vi "message handler main.vi"(11 "messageHandler":T2 {"params"."controlChannels"."ballControl" items=["Module6/output0", "Module6/output1", "Module6/output2", "Module6/output3", "Not-Used"]; "params"."controlChannels"."butterflyControl" items=["Module6/output0", "Module6/output1", "Module6/output2", "Module6/output3", "Not-Used"]; "params"."controlChannels"."speedControl" items=["Module6/output0", "Module6/output1", "Module6/output2", "Module6/output3", "Not-Used"]}) -> ()   [LabVIEW 2018]
uses:
  supporting VIs/polymorphic VIs/enqueue for data stream.vi
  supporting VIs/polymorphic VIs/enqueue for comms.vi
  supporting VIs/polymorphic VIs/enqueue for user interface.vi
  RT/Type Defs/RT Status.ctl
  supporting VIs/polymorphic VIs/enqueue for custom.vi
  supporting VIs/polymorphic VIs/release message handler queue.vi
  supporting VIs/polymorphic VIs/enqueue for message handler.vi
  supporting VIs/polymorphic VIs/de-queue for message handler.vi
  supporting VIs/polymorphic VIs/enqueue for data processor.vi
  comms loop/delayedMessages/delayedMessageHandler.vi
  customVI/liveData/state.ctl
  type defs/message handler data.ctl
panel:
  out "RT status":T1
  out "commands":string[](array[string])
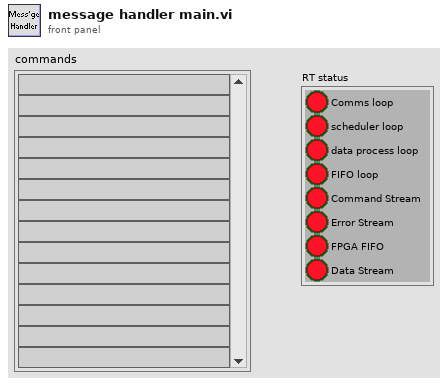
[diagram p1: front panel]
types:
  T1 = typedef "RT Status.ctl" = cluster{"Comms loop":bool, "scheduler loop":bool, "data process loop":bool, "FIFO loop":bool, "Command Stream":bool, "Error Stream":bool, "FPGA FIFO":bool, "Data Stream":bool}
  T2 = typedef "message handler data.ctl" = cluster{"params":cluster{"configFileID":u32, "configFilePath":path, "channelConfigFilePath":path, "incidentLogfile":path, "controlChannels":cluster{"ballControl":u16, "butterflyControl":u16, "speedControl":u16}, "pulsatorVIPath":path, "customVIPath":path, "HowdenAir":cluster{"vent Howden":bool, "Howden%":dbl}}, "vars":cluster{"commsStatus":bool[], "controlIndex":cluster{"ballControl":u16, "butterflyControl":u16, "speedControl":u16}, "customVIRef":refnum<vi>, "Interlocks":cluster{"gearboxOil":bool, "bearingOil":bool, "gearboxAir":bool}, "motorRunning":bool, "liveDataQ":refnum<queue>[]}}
  T3 = typedef "Queues.ctl" = cluster{"messageHandler":refnum<queue>, "comms":refnum<queue>, "dataStream":refnum<queue>, "dataProcessor":refnum<queue>, "fileIO":refnum<queue>, "userInterface":refnum<queue>, "errors":refnum<queue>, "customCompressor":refnum<queue>}
  T4 = cluster{"gearboxOil":bool, "bearingOil":bool, "gearboxAir":bool}
  T5 = typedef "state.ctl" = enum16{"readData", "init", "channel", "mode", "quit"}
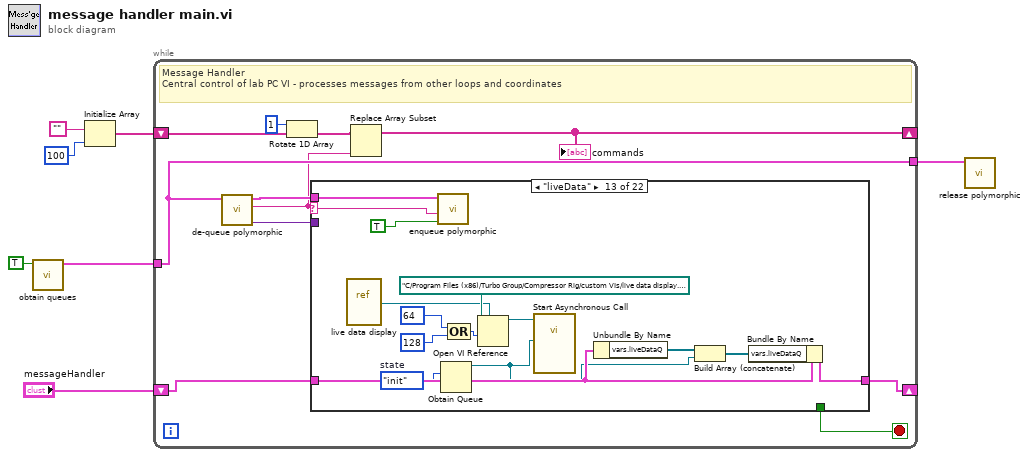
[diagram p0: block diagram]
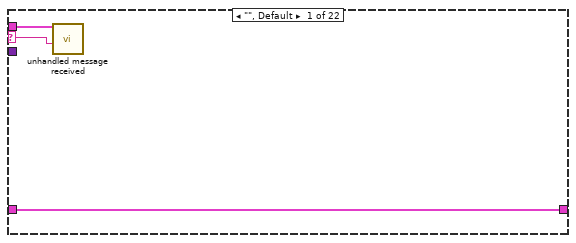
[diagram p2: hidden frame]
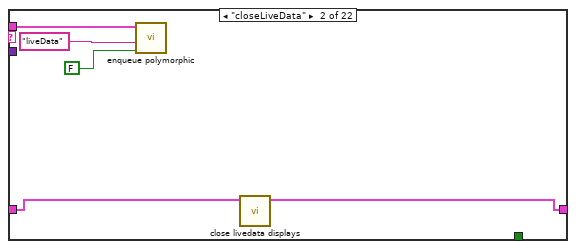
[diagram p3: hidden frame]
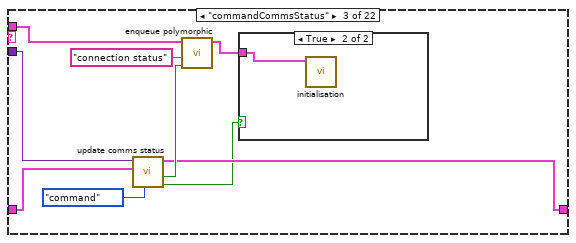
[diagram p4: hidden frame]
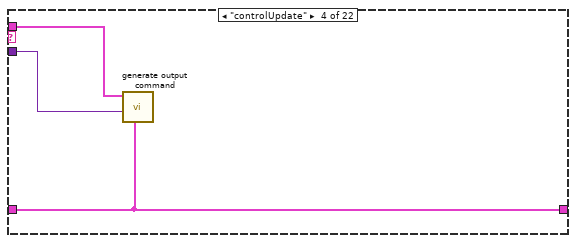
[diagram p6: hidden frame]
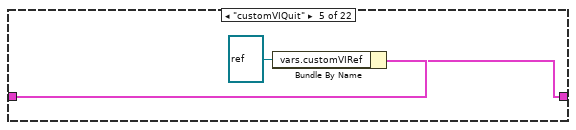
[diagram p7: hidden frame]
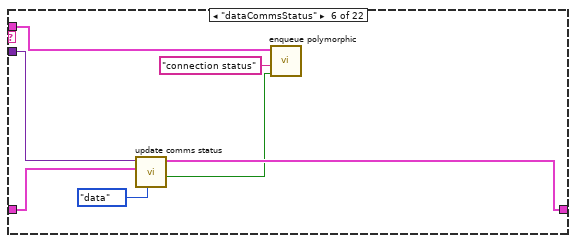
[diagram p8: hidden frame]
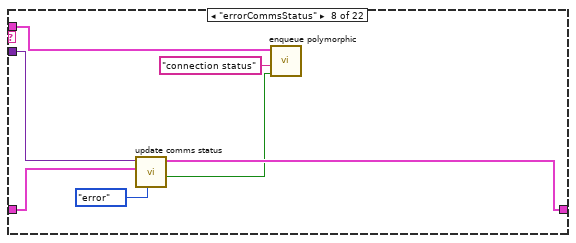
[diagram p10: hidden frame]
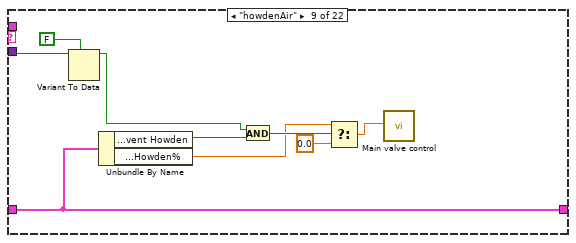
[diagram p11: hidden frame]
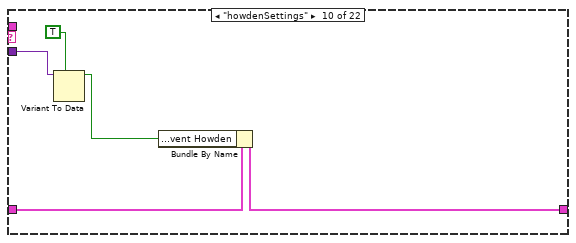
[diagram p12: hidden frame]
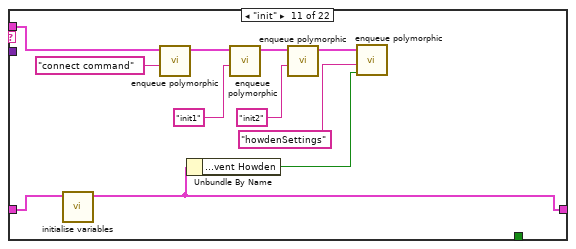
[diagram p13: hidden frame]
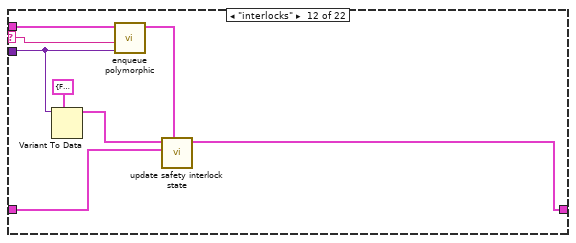
[diagram p14: hidden frame]
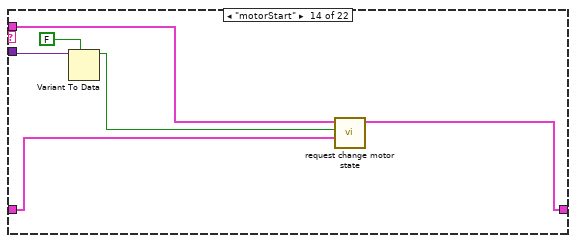
[diagram p15: hidden frame]
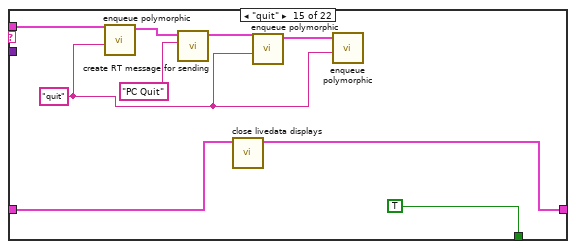
[diagram p16: hidden frame]
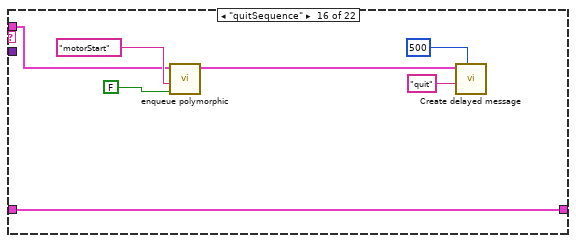
[diagram p17: hidden frame]
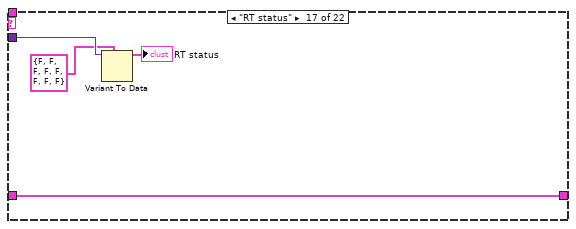
[diagram p18: hidden frame]
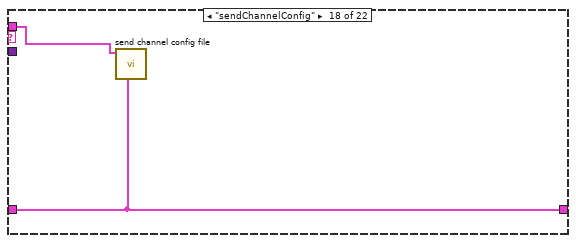
[diagram p19: hidden frame]
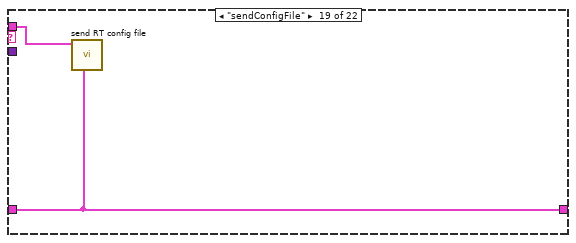
[diagram p20: hidden frame]
diagram:
  n1 = call "obtain queues.vi"("initialise? (F)"=TRUE) -> ("queues"=w7:T3)  [unwired: 10 in]
  n2 = Initialize Array("", 100 ("dimension size")) -> (w3:string[])
  n3 = while {
    tunnel: w7 -> [w15]
    tunnel: [w15] -> w6
    shift-right: [w14] -> _
    shift-left: "messageHandler" -> [w13]
    shift-right: [w9] -> _
    shift-left: w3 -> [w12]
    stop <- w17 stop-if-true
    # "Message Handler\nCentral control of lab PC VI - processes messages from other loops and coordinates"
    n4 = call-poly "de-queue polymorphic.vi"("Queues"=w15) -> ("data"=w18:variant, "message"=w8:string, "Queues out"=w16:T3)  [unwired: 8 in]
    n5 = Rotate 1D Array(1:w12, 2:1 ("n")) -> (0:w10:string[])
    n6 = case shown="\"liveData\"" w8 {
      selector: w8 -> [w19 _ _ _ _ _ _ _ _ _ _ w88 w100 _ _ _ _ _ _ _ _ _]
      tunnel: w18 -> [_ _ w34 w38 _ w47 _ w55 w66 w69 _ w86 _ w111 _ _ w131 _ _ _ w141 _]
      tunnel: [_ _ _ _ _ _ _ _ _ _ _ _ _ _ TRUE _ _ _ _ _ _ _] -> w17
      tunnel: w16 -> [w20 w26 w32 w39 _ w45 _ w53 _ _ w80 w89 w101 w109 w114 w125 _ w133 w135 w138 w140 _]
      tunnel: [w21 w24 w28 w37 w41 w48 w50 w56 w64 w70 w73 w87 w98 w107 w112 w124 w128 w132 w134 w136 w139 w142] -> w14
      tunnel: w13 -> [w21 w25 w35 w37 w42 w49 w50 w57 w64 w71 w82 w90 w99 w108 w113 w124 w128 w132 w134 w137 w139 w142]
      frame "", Default {
        n7 = call "unhandled message received.vi"("unhandledMessage"=w19, "queues"=w20) -> ()  [unwired: 10 in]
      }
      frame "closeLiveData" {
        n8 = call-poly "enqueue polymorphic.vi"("data"=FALSE, "message"="liveData", "Queues"=w26) -> ()  [unwired: 8 in, 1 out]
        n9 = call "close livedata displays.vi"("messageHandler in"=w25) -> ("messageHandler out"=w24:T2)  [unwired: 10 in]
      }
      frame "commandCommsStatus" {
        n10 = call "update comms status.vi"("comms"=enum16{"command", "error", "data"}."command", "messageHandler in"=w35, "data"=w34) -> ("this comms"=w27:bool, "connection status"=w30:bool, "messageHandler out"=w28:T2)  [unwired: 6 in]
        n11 = call-poly "enqueue polymorphic.vi"("data"=w30, "message"="connection status", "Queues"=w32) -> ("Queues out"=w29:T3)  [unwired: 8 in]
        n12 = case shown="True" w27 {
          tunnel: w29 -> [_ w36]
          frame False {
          }
          frame True {
            n13 = call "initialisation.vi"("Queues in"=w36) -> ()  [unwired: 11 in]
          }
        }
      }
      frame "controlUpdate" {
        n14 = call "generate output command.vi"("messageHandler"=w37, "control data"=w38, "Queues in"=w39) -> ()  [unwired: 9 in]
      }
      frame "customVIQuit" {
        n15 = Bundle By Name(cluster=w42, "vars.customVIRef"=refnum<vi> refnum) -> (w41:T2)
      }
      frame "dataCommsStatus" {
        n16 = call "update comms status.vi"("comms"=enum16{"command", "error", "data"}."data", "messageHandler in"=w49, "data"=w47) -> ("connection status"=w43:bool, "messageHandler out"=w48:T2)  [unwired: 6 in, 1 out]
        n17 = call-poly "enqueue polymorphic.vi"("data"=w43, "message"="connection status", "Queues"=w45) -> ()  [unwired: 8 in, 1 out]
      }
      frame "error received" {
      }
      frame "errorCommsStatus" {
        n18 = call "update comms status.vi"("comms"=enum16{"command", "error", "data"}."error", "messageHandler in"=w57, "data"=w55) -> ("connection status"=w51:bool, "messageHandler out"=w56:T2)  [unwired: 6 in, 1 out]
        n19 = call-poly "enqueue polymorphic.vi"("data"=w51, "message"="connection status", "Queues"=w53) -> ()  [unwired: 8 in, 1 out]
      }
      frame "howdenAir" {
        n20 = Variant To Data(type=FALSE ("new output"), Variant=w66) -> (data=w62:bool)  [unwired: 1 in, 1 out]
        n21 = Unbundle By Name(w64) -> ("params.HowdenAir.vent Howden"=w63:bool, "params.HowdenAir.Howden%"=w60:dbl)
        n22 = And(x=w62, y=w63) -> (x .and. y?=w61:bool)
        n23 = Select(t=w60, s=w61, f=0.0) -> (s? t:f=w58:dbl)
        n24 = call "Main valve control.vi"("Main Valve (%)"=w58) -> ()  [unwired: 9 in, 2 out]
      }
      frame "howdenSettings" {
        n25 = Variant To Data(type=TRUE, Variant=w69) -> (data=w68:bool)  [unwired: 1 in, 1 out]
        n26 = Bundle By Name(cluster=w71, "params.HowdenAir.vent Howden"=w68) -> (w70:T2)
      }
      frame "init" {
        n27 = call "initialise variables.vi"("messageHandler in"=w82) -> ("messageHandler out"=w73:T2)  [unwired: 10 in]
        n28 = call-poly "enqueue polymorphic.vi"("message"="connect command", "Queues"=w80) -> ("Queues out"=w79:T3)  [unwired: 9 in]
        n29 = Unbundle By Name(w73) -> ("params.HowdenAir.vent Howden"=w72:bool)
        n30 = call-poly "enqueue polymorphic.vi"("message"="init1", "Queues"=w79) -> ("Queues out"=w77:T3)  [unwired: 9 in]
        n31 = call-poly "enqueue polymorphic.vi"("message"="init2", "Queues"=w77) -> ("Queues out"=w75:T3)  [unwired: 9 in]
        n32 = call-poly "enqueue polymorphic.vi"("data"=w72, "message"="howdenSettings", "Queues"=w75) -> ()  [unwired: 8 in, 1 out]
      }
      frame "interlocks" {
        n33 = Variant To Data(type=T4 {"gearboxOil"=FALSE, "bearingOil"=FALSE, "gearboxAir"=FALSE} ("vars.Interlocks"), Variant=w86) -> (data=w84:T4)  [unwired: 1 in, 1 out]
        n34 = call-poly "enqueue polymorphic.vi"("data"=w86, "message"=w88, "Queues"=w89) -> ("Queues out"=w83:T3)  [unwired: 8 in]
        n35 = call "update safety interlock state.vi"("queues"=w83, "messageHandler in"=w90, "vars.Interlocks"=w84) -> ("messageHandler out"=w87:T2)  [unwired: 8 in]
      }
      frame "liveData" {
        w93 = state."init"  # state
        n36 = vi-ref "live data display.vi"() -> (w102:refnum<vi>)
        n37 = call-poly "enqueue polymorphic.vi"("data"=TRUE, "message"=w100, "Queues"=w101) -> ()  [unwired: 8 in, 1 out]
        n38 = Obtain Queue(element data type=w93) -> (queue out=w91:refnum<queue>)  [unwired: 4 in, 2 out]
        n39 = Compound Arithmetic op=OR(64 ("options"), 128 ("options")) -> (w95:i32)
        n40 = Open VI Reference(type specifier VI Refnum (for type only)=w102, vi path=path "C:/Program Files (x86)/Turbo Group/Compressor Rig/custom VIs/live data display.vi", options=w95) -> (vi reference=w103:refnum<vi>)  [unwired: 3 in, 1 out]
        n41 = call-by-ref "Start Asynchronous Call"(reference=w103, "queue"=w91) -> ()  [unwired: 12 in, 2 out]
        n42 = Unbundle By Name(w99) -> ("vars.liveDataQ"=w97:refnum<queue>[])
        n43 = Build Array (concatenate)(w97, w91) -> (w92:refnum<queue>[])
        n44 = Bundle By Name(cluster=w99, "vars.liveDataQ"=w92) -> (w98:T2)
      }
      frame "motorStart" {
        n45 = Variant To Data(type=FALSE ("new output"), Variant=w111) -> (data=w106:bool)  [unwired: 1 in, 1 out]
        n46 = call "request change motor state.vi"("messageHandler in"=w108, "new output"=w106, "Queues in"=w109) -> ("messageHandler out"=w107:T2)  [unwired: 8 in]
      }
      frame "quit" {
        w115 = "quit" ("message")
        n47 = call-poly "enqueue polymorphic.vi"("message"=w115, "Queues"=w114) -> ("Queues out"=w118:T3)  [unwired: 9 in]
        n48 = call "create RT message for sending.vi"("RT message"="PC Quit", "Queues in"=w118) -> ("Queues out"=w117:T3)  [unwired: 9 in]
        n49 = call "close livedata displays.vi"("messageHandler in"=w113) -> ("messageHandler out"=w112:T2)  [unwired: 10 in]
        n50 = call-poly "enqueue polymorphic.vi"("message"=w115, "Queues"=w117) -> ("Queues out"=w116:T3)  [unwired: 9 in]
        n51 = call-poly "enqueue polymorphic.vi"("message"=w115, "Queues"=w116) -> ()  [unwired: 9 in, 1 out]
      }
      frame "quitSequence" {
        n52 = call-poly "enqueue polymorphic.vi"("data"=FALSE ("QUIT"), "message"="motorStart", "Queues"=w125) -> ("Queues out"=w123:T3)  [unwired: 8 in]
        n53 = call-poly "Create delayed message.vi"("ms delay"=u32 500, "message"="quit", "Queues in"=w123) -> ()  [unwired: 9 in]
      }
      frame "RT status" {
        n54 = Variant To Data(type=T1 {"Comms loop"=FALSE, "scheduler loop"=FALSE, "data process loop"=FALSE, "FIFO loop"=FALSE, "Command Stream"=FALSE, "Error Stream"=FALSE, "FPGA FIFO"=FALSE, "Data Stream"=FALSE} ("RT Status"), Variant=w131) -> (data=→"RT status":T1)  [unwired: 1 in, 1 out]
      }
      frame "sendChannelConfig" {
        n55 = call "send channel config file.vi"("messageHandler"=w132, "Queues"=w133) -> ()  [unwired: 10 in]
      }
      frame "sendConfigFile" {
        n56 = call "send RT config file.vi"("messageHandler"=w134, "Queues"=w135) -> ()  [unwired: 10 in]
      }
      frame "start customVI" {
        n57 = call "launch custom VI.vi"("messageHandler in"=w137, "Queues in"=w138) -> ("messageHandler out"=w136:T2)  [unwired: 9 in]
      }
      frame "updateChannelConfig" {
        n58 = call "update channel config path in user config.vi"("messageHandler in"=w139, "new path"=w141, "Queues in"=w140) -> ()  [unwired: 9 in]
      }
      frame "warning received" {
      }
    }
    n59 = Replace Array Subset(array=w10, new element=w8) -> (w9:string[])  [unwired: 1 in]
    "commands" <- w9
  }
  n60 = call-poly "release polymorphic.vi"("Queues"=w6) -> ()  [unwired: 11 in]
